vi "LinxDigitalRead.vi"(8 "Error In":errorcluster, 10 "Channels":u8[](array[numeric]), 11 "LINX Resource":T1) -> (0 "Error Out":errorcluster, 2 "Values":bool[](array[boolean]), 3 "LINX Resource":T1)   [LabVIEW 2014, in "LMH-LINX.lvlib" / "Local IO.lvlib"]
uses:
  Local IO.lvlib
  Type Defs/LINX Ref.ctl
  Type Defs/Platform.ctl
  Type Defs/Interface.ctl
  Device/Type Defs/LINX Device Config.ctl
  Device/Type Defs/TCP Config.ctl
  Device/Type Defs/Channels.ctl
  <vilib>/myRIO/Instrument Drivers/Onboard IO/DIO/DIO.lvlib
  myRIO/myRIO.lvlib
  liblinxdevice.dll
  LMH-LINX.lvlib
  Device/Device.lvlib
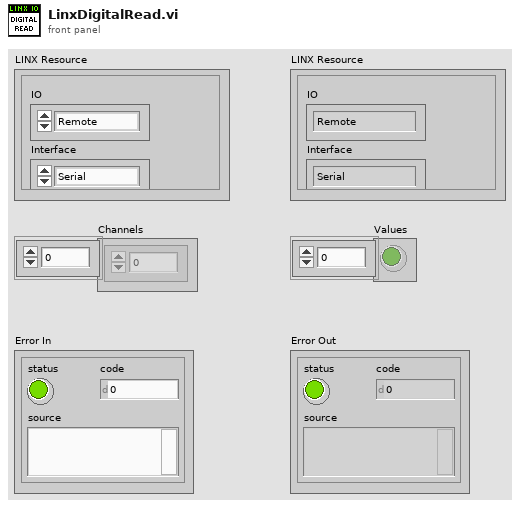
[diagram p1: front panel]
types:
  T1 = typedef "LMH-LINX.lvlib/LINX Ref.ctl" = cluster{"IO":T2, "Interface":T3, "LINX Device Config":T4}
  T2 = typedef "LMH-LINX.lvlib/Platform.ctl" = enum16{"Remote", "Local"}
  T3 = typedef "LMH-LINX.lvlib/Interface.ctl" = enum16{"Serial", "TCP"}
  T4 = typedef "LMH-LINX.lvlib/Device.lvlib/LINX Device Config.ctl" = cluster{"Interface":T3, "COM Port":refnum<visa-resource-name>, "TCP Configuration":T5, "Device Family":u8, "Device ID":u8, "Device Name":string, "TCP Ref":refnum<k5>, "Channels":T6}
  T5 = typedef "LMH-LINX.lvlib/Device.lvlib/TCP Config.ctl" = cluster{"IP Address":string, "Port":u16}
  T6 = typedef "LMH-LINX.lvlib/Channels.ctl" = cluster{"DI":u8[], "DO":u8[], "AI":u8[], "AO":u8[], "PWM":u8[], "QE":u8[], "UART":u8[], "I2C 2":u8[], "SPI":u8[], "CAN":u8[], "Servo":u8[], "AI Ref (V)":dbl, "AI Resolution (Bits)":u8, "AO Ref (V)":dbl, "AO Resolution (Bits)":u8}
  T7 = typedef "DIO.lvlib/DIO Reference.ctl" = cluster{"myRIO Reference":T8, "DIO Channels List":T12}
  T8 = typedef "myRIO Generic Hardware Reference.ctl" = cluster{"myRIO Model":T9, "myRIO Hardware Reference":T10}
  T9 = typedef "Hardware Version Enum.ctl" = enum16{"Unknown", "myRIO-1900", "myRIO-1950"}
  T10 = typedef "myRIO v1.0 Reference.ctl" = cluster{"Generic FPGA Reference":T11, "Allow multiple opens":bool}
  T11 = typedef "Generic FPGA Reference.ctl" = refnum<k20>
  T12 = typedef "DIO Channels List.ctl" = T13[]
  T13 = typedef "DIO Channels Enum.ctl" = enum16{"Not Connected", "C/DIO0", "C/DIO1", "C/DIO2", "C/DIO3", "C/DIO4", "C/DIO5", "C/DIO6", "C/DIO7", "A/DIO0", "A/DIO1", "A/DIO2", "A/DIO3", "A/DIO4", "A/DIO5", "A/DIO6", "A/DIO7", "A/DIO8", "A/DIO9", "A/DIO10", "A/DIO11", "A/DIO12", "A/DIO13", "A/DIO14", "A/DIO15", "B/DIO0", "B/DIO1", "B/DIO2", "B/DIO3", "B/DIO4", "B/DIO5", "B/DIO6", "B/DIO7", "B/DIO8", "B/DIO9", "B/DIO10", "B/DIO11", "B/DIO12", "B/DIO13", "B/DIO14", "B/DIO15", "LED0", "LED1", "LED2", "LED3", "Button0"}
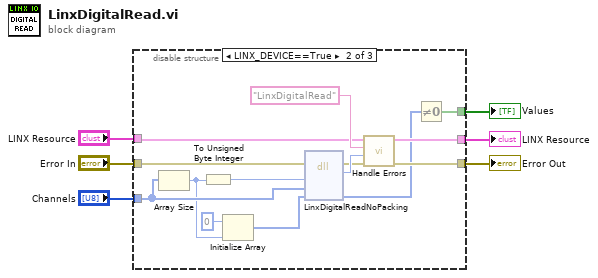
[diagram p0: block diagram]
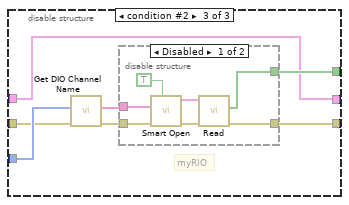
[diagram p3: hidden frame]
diagram:
  n1 = disable-structure shown="LINX_DEVICE==True" {
    disable-tunnel: [w8 w17 w23] -> w6
    disable-tunnel: [w7 w16 w25] -> w5
    disable-tunnel: "LINX Resource" -> [w8 w14 w23]
    disable-tunnel: "Error In" -> [w7 w15 w26]
    disable-tunnel: "Channels" -> [_ w13 w27]
    disable-tunnel: [_ w9 w24] -> w1
    frame condition #0 (active) {
    }
    frame condition #1 {
      n2 = Array Size(array=w13) -> (size(s)=w12:i32)
      n3 = To Unsigned Byte Integer(number=w12) -> (unsigned 8bit integer=w11:u8)
      n4 = Initialize Array(u8 0 ("element"), w12) -> (w22:u8[])
      n5 = dll-call lib="liblinxdevice.*" fn="LinxDigitalReadNoPacking"(error in=w15, "numChans"=w11, "channels"=w13, "values"=w22) -> (error out=w18:errorcluster, "LinxStatus"=w19:i32, "values"=w10:u8[])  [unwired: 4 in, 1 out]
      n6 = call "Handle Errors.vi"("Error In"=w18, "LinxStatus"=w19, "Function Name"="LinxDigitalRead", "LINX Resource"=w14) -> ("Error Out"=w16:errorcluster, "LINX Resource"=w17:T1)  [unwired: 6 in]
      n7 = Not Equal To 0?(x=w10) -> (x != 0?=w9:bool[])
    }
    frame condition #2 {
      # "myRIO"
      n8 = call "Get DIO Channel Name.vi"("Error In"=w26, "DIO Channel Nums"=w27) -> ("Error Out"=w28:errorcluster, "DIO Channels"=w29:string[])  [unwired: 8 in]
      n9 = disable-structure shown="Disabled" {
        disable-tunnel: [w36 _] -> w25
        disable-tunnel: w28 -> [w34 _]
        disable-tunnel: w29 -> [w35 _]
        disable-tunnel: [w30 _] -> w24
        frame Disabled {
          n10 = call <vilib>:"Smart Open.vi"("Allow multiple opens?"=TRUE, "error in (no error)"=w34, "Channel Names"=w35) -> ("error out"=w33:errorcluster, "DIO Ref Out"=w32:T7)  [unwired: 7 in]
          n11 = call <vilib>:"Read.vi"("error in (no error)"=w33, "DIO Ref In"=w32) -> ("error out"=w36:errorcluster, "Values"=w30:bool[])  [unwired: 7 in, 1 out]
        }
        frame Enabled {
        }
      }
    }
  }
  "Error Out" <- w5
  "LINX Resource" <- w6
  "Values" <- w1
